vi "VariableDelete.vi"(8 "error in (no error)":errorcluster, 10 "VariableName":string, 11 "VariableManagerRef in":refnum<vi>) -> (0 "error out":errorcluster, 3 "VariableManagerRef out":refnum<vi>)   [LabVIEW 2013, in "VariableManagerAPI.lvlib"]
doc: "Delete VariableName from database. \nNo operation if VariableName does not exist"
uses:
  VariableManagerAPI.lvlib
  VariableManager/VariableManager.lvclass
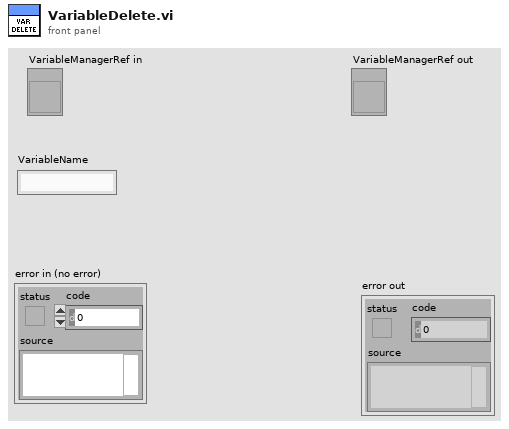
[diagram p1: front panel]
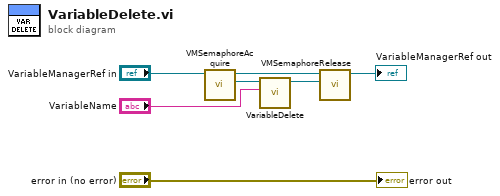
[diagram p0: block diagram]
diagram:
  n1 = call "VMSemaphoreAcquire.vi"("VariableManagerRef in"="VariableManagerRef in") -> ("VariableManager"=w3:refnum<class "VariableManager.lvclass">, "VariableManagerRef out"=w6:refnum<vi>)  [unwired: 7 in, 2 out]
  n2 = call-dynamic "VariableDelete.vi"("VariableName"="VariableName", "VariablesManager in"=w3) -> ("VariablesManager out"=w2:refnum<class "VariableManager.lvclass">)  [unwired: 8 in, 1 out]
  n3 = call "VMSemaphoreRelease.vi"("VariableManager"=w2, "VariableManagerRef in"=w6) -> ("VariableManagerRef out"=→"VariableManagerRef out":refnum<vi>)  [unwired: 8 in, 1 out]
  "error out" <- "error in (no error)"
